vi "Q_Get Leaderboard by Athlete and Type.vi"(8 "error in (no error)":errorcluster, 11 "Data Manager in":refnum<class "Data Manager.lvclass">) -> (0 "error out":errorcluster, 2 "All Tables":T1(array[cluster]), 3 "Data Manager out":refnum<class "Data Manager.lvclass">)   [LabVIEW 2020, in "Data Manager.lvclass"]
uses:
  Data Manager.lvclass
  Data Manager.lvclass/Data Manager.ctl
  <vilib>/drjdpowell/SQLite Library/SQL Connection/Execute SQL.vi
  <vilib>/drjdpowell/SQLite Library/SQLite.lvlib
  <vilib>/drjdpowell/SQLite Library/SQL Connection/Connection.lvclass
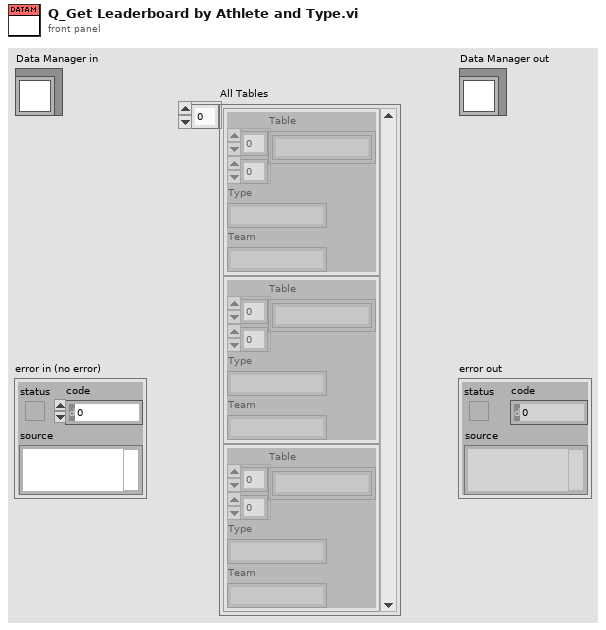
[diagram p1: front panel]
types:
  T1 = cluster{"Table":string[][], "Type":string, "Team":string}[]
  T2 = typedef "Data Manager.lvclass/Name--cluster.ctl" = cluster{"First":string, "Last":string}
  T3 = typedef "Data Manager.lvclass/Profile--cluster.ctl" = cluster{"Alias":string, "Team":string}
  T4 = cluster{"Table":string[][], "Type":string, "Team":string}
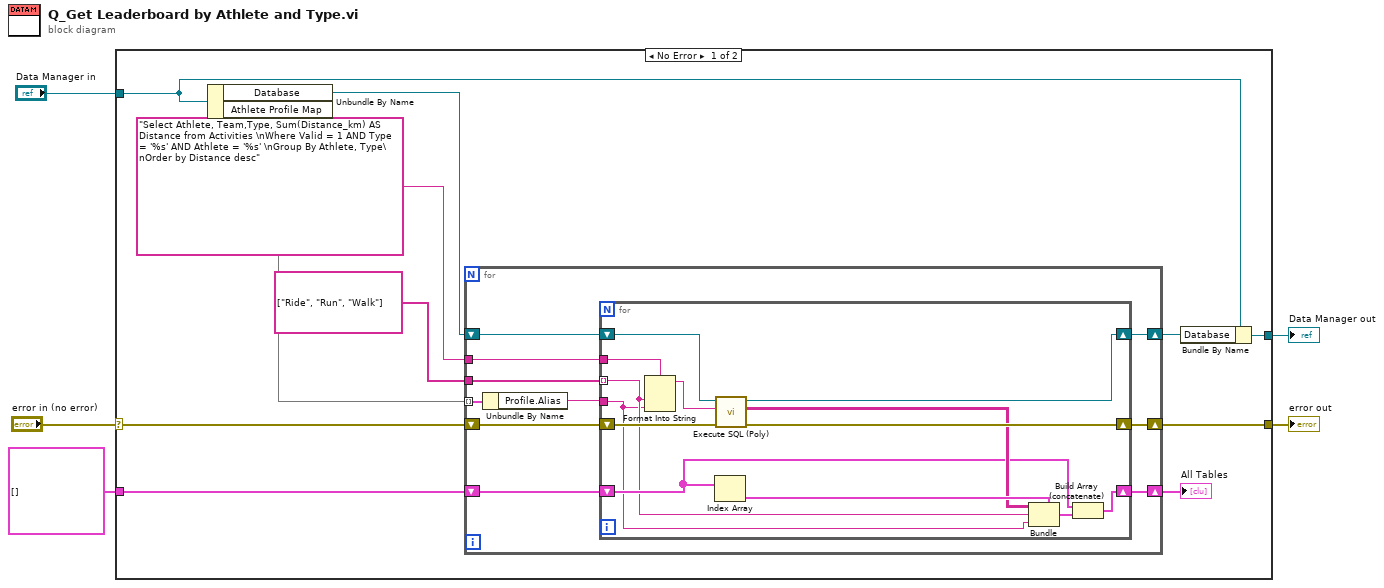
[diagram p0: block diagram]
diagram:
  n1 = case shown="No Error" "error in (no error)" {
    selector: "error in (no error)" -> [w12 w41]
    tunnel: [w11 w41] -> w4
    tunnel: [w14 w40] -> w2
    tunnel: "Data Manager in" -> [w15 w40]
    tunnel: T1 [] ("All Tables") -> [w8 _]
    frame No Error {
      n2 = Unbundle By Name(w15) -> ("Database"=w16:refnum<class "Connection.lvclass">, "Athlete Profile Map"=w6:map{T2, T3})
      n3 = for {
        tunnel: "Select Athlete, Team,Type, Sum(Distance_km) AS Distance from Activities \nWhere Valid = 1 AND Type = '%s' AND Athlete = '%s' \nGroup By Athlete, Type\nOrder by Distance desc" ("SQL") -> [w22]
        shift-right: [w25] -> w13
        shift-left: w16 -> [w26]
        shift-right: [w23] -> w11
        shift-left: w12 -> [w24]
        tunnel: string[] ["Ride", "Run", "Walk"] -> [w21]
        tunnel: w6 -> [w18] mode=indexing
        shift-right: [w19] -> w7
        shift-left: w8 -> [w20]
        n4 = Unbundle By Name(w18) -> ("Profile.Alias"=w17:string)
        n5 = for {
          tunnel: w22 -> [w35]
          shift-right: [w38] -> w25
          shift-left: w26 -> [w39]
          shift-right: [w36] -> w23
          shift-left: w24 -> [w37]
          tunnel: w21 -> [w28] mode=indexing
          tunnel: w17 -> [w27]
          shift-right: [w30] -> w19
          shift-left: w20 -> [w29]
          n6 = Format Into String(format string=w35, w28, w27) -> (resulting string=w34:string)  [unwired: 2 in, 1 out]
          n7 = Index Array(array=w29) -> (element=w33:T4)  [unwired: 1 in]
          n8 = call-poly <vilib>:"Execute SQL (Poly).vi"("error in (no error)"=w37, "SQL"=w34, "SQLite Connection in"=w39) -> ("error out"=w36:errorcluster, "Result Set"=w32:string[][], "SQLite Connection"=w38:refnum<class "Connection.lvclass">)  [unwired: 5 in, 1 out]
          n9 = Bundle(cluster=w33, "Table"=w32, "Type"=w28, "Team"=w27) -> (w31:T4)
          n10 = Build Array (concatenate)(w29, w31) -> (w30:T1)
        }
      }
      "All Tables" <- w7
      n11 = Bundle By Name(cluster=w15, "Database"=w13) -> (w14:refnum<class "Data Manager.lvclass">)
    }
    frame Error {
    }
  }
  "error out" <- w4
  "Data Manager out" <- w2
